vi "ZDataVIS_EstSize_(mb).vi"(10 "1D arrays":dbl[][](array[numeric]), 11 "Numeric":i32) -> (3 "total megabyte estimate":dbl=72.479248046875)   [LabVIEW 2016]
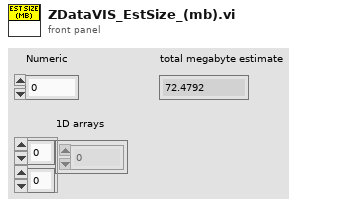
[diagram p1: front panel]
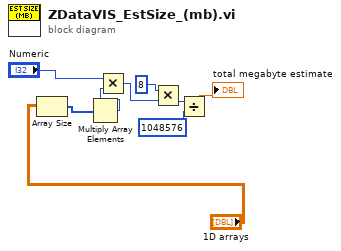
[diagram p0: block diagram]
diagram:
  n1 = Array Size(array="1D arrays") -> (size(s)=w2:i32[])
  n2 = Multiply Array Elements(1:w2) -> (0:w4:i32)
  n3 = Multiply(x="Numeric", y=w4) -> (x*y=w5:i32)
  n4 = Multiply(x=8, y=w5) -> (x*y=w7:i32)
  n5 = Divide(x=w7, y=1048576) -> (x/y=→"total megabyte estimate":dbl)
